vi "Parse REST Device Readings.vi"(3 "error in (no error)":errorcluster, 5 "Reading XML":string="<?xml version=\"1.0\" encoding=\"ISO-8859-1\" standalone=\"no\" ?>\n<methodResponse>\n\n  <params>\n    <param>\n      <value>\n        <struct>\n          <member>\n            <name>status</name>\n            <value>\n              <int>0</int>\n            </value>\n          </member>\n          <member>\n            <name>scaled</name>\n            <value>\n              <double>0.9992975666172701</double>\n            </value>\n          </member>\n          <member>\n            <name>units</name>\n            <value>Torr</value>\n          </member>\n          <member>\n            <name>name</name>\n            <value>e:201vac</value>\n          </member>\n        </struct>\n      </value>\n    </param>\n  </params>\n\n</methodResponse>\n") -> (0 "error out":errorcluster, 1 "Pending":bool, 2 "ACNET Device Readings":T1(array[cluster]))   [LabVIEW 2013]
uses:
  <vilib>/xml/Close Reference(Node).vi
  <vilib>/xml/Close Reference(NdList).vi
  <vilib>/xml/NI_XML.lvlib
  <resource>/objmgr/DOMUserDefRef.rc
panel:
  out "Parse Errors":string
  out "XML Response":string
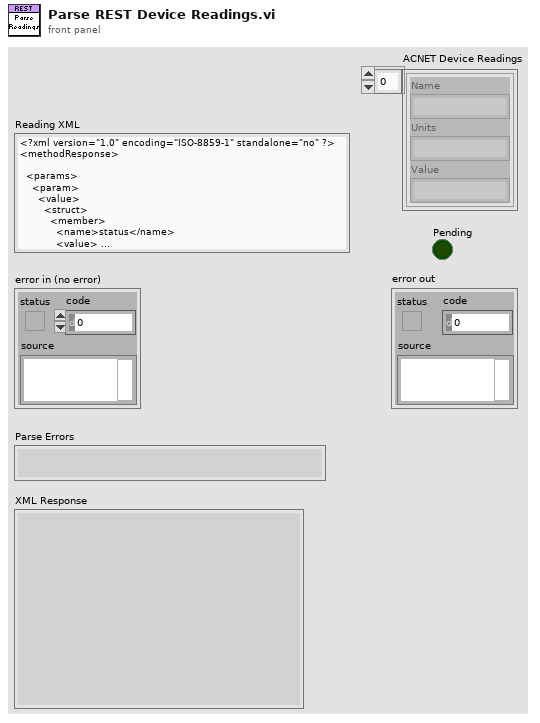
[diagram p1: front panel]
types:
  T1 = cluster{"Name":string, "Units":string, "Value":string}[]
  T2 = cluster{"Name":string, "Units":string, "Value":string}
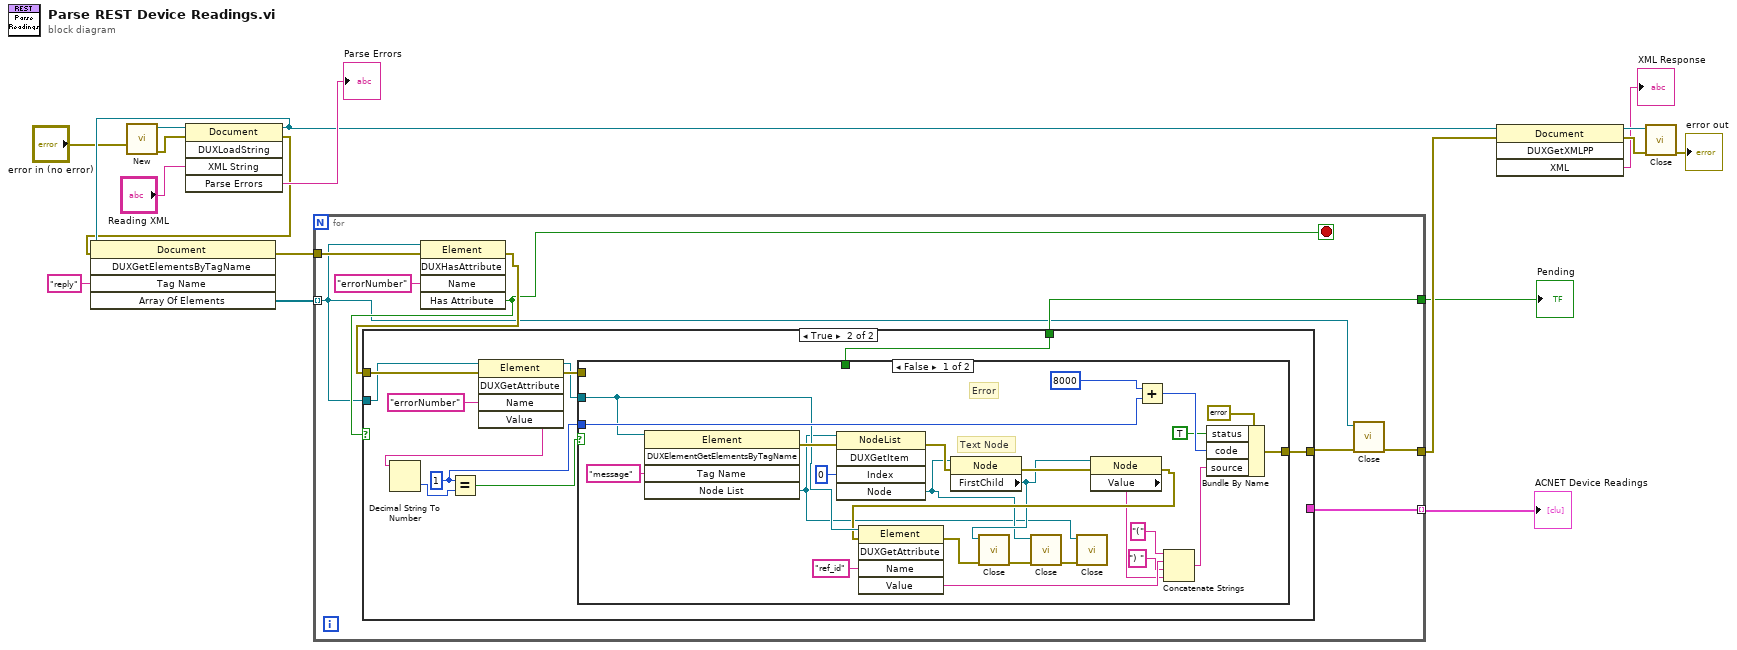
[diagram p0: block diagram]
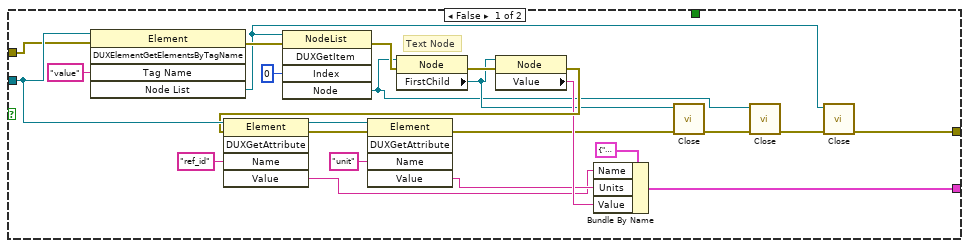
[diagram p2: hidden frame]
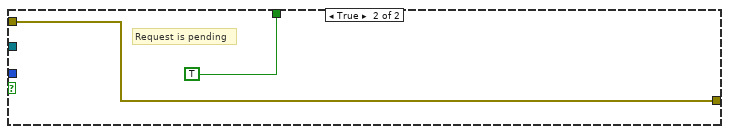
[diagram p3: hidden frame]
diagram:
  n1 = call <vilib>:"New.vi"("error in (no error)"="error in (no error)") -> ("error out"=w13:errorcluster, "DOM document out"=w12:refnum<k20>)  [unwired: 7 in]
  n2 = invoke class="Document" method="DUXLoadString"(reference=w12, error in=w13, "XML String"="Reading XML") -> (reference out=w9:refnum<k20>, error out=w8:errorcluster, "Parse Errors"=→"Parse Errors":string)  [unwired: 2 in, 2 out]
  n3 = invoke class="Document" method="DUXGetElementsByTagName"(reference=w9, error in=w8, "Tag Name"="reply") -> (error out=w6:errorcluster, "Array Of Elements"=w7:refnum<k20>[])  [unwired: 2 in, 3 out]
  n4 = for {
    tunnel: w7 -> [w18] mode=indexing
    tunnel: w6 -> [w26]
    tunnel: [w23] -> w3 mode=indexing
    tunnel: [w21] -> w1
    tunnel: [w20] -> w2
    stop <- w22 stop-if-true
    n5 = invoke class="Element" method="DUXHasAttribute"(reference=w18, error in=w26, "Name"="errorNumber") -> (error out=w24:errorcluster, "Has Attribute"=w22:bool)  [unwired: 2 in, 3 out]
    n6 = case shown="True" w22 {
      tunnel: w18 -> [w48 w58]
      tunnel: w24 -> [w47 w59]
      tunnel: [w33 w54] -> w19
      tunnel: [w34 _] -> w23
      tunnel: [_ w53] -> w21
      frame False {
        # "Text Node"
        n7 = invoke class="Element" method="DUXElementGetElementsByTagName"(reference=w48, error in=w47, "Tag Name"="value") -> (error out=w41:errorcluster, "Node List"=w30:refnum<k20>)  [unwired: 2 in, 3 out]
        n8 = invoke class="NodeList" method="DUXGetItem"(reference=w30, error in=w41, "Index"=0) -> (error out=w39:errorcluster, "Node"=w27:refnum<k20>)  [unwired: 2 in, 3 out]
        n9 = property class="Node"(reference=w27, error in=w39) -> (error out=w49:errorcluster, "FirstChild"=w31:refnum<k20>)  [unwired: 1 out]
        n10 = property class="Node"(reference=w31, error in=w49) -> (error out=w44:errorcluster, "Value"=w37:string)  [unwired: 1 out]
        n11 = invoke class="Element" method="DUXGetAttribute"(reference=w48, error in=w44, "Name"="ref_id") -> (reference out=w43:refnum<k20>, error out=w42:errorcluster, "Value"=w35:string)  [unwired: 2 in, 2 out]
        n12 = invoke class="Element" method="DUXGetAttribute"(reference=w43, error in=w42, "Name"="unit") -> (error out=w32:errorcluster, "Value"=w36:string)  [unwired: 2 in, 3 out]
        n13 = Bundle By Name(cluster=T2 {"Name"="", "Units"="", "Value"=""}, "Name"=w35, "Units"=w36, "Value"=w37) -> (w34:T2)
        n14 = call-poly <vilib>:"Close.vi"("error in (no error)"=w32, "node"=w31) -> ("error out"=w29:errorcluster)  [unwired: 7 in]
        n15 = call-poly <vilib>:"Close.vi"("error in (no error)"=w29, "node"=w27) -> ("error out"=w28:errorcluster)  [unwired: 7 in]
        n16 = call-poly <vilib>:"Close.vi"("error in (no error)"=w28, "node list"=w30) -> ("error out"=w33:errorcluster)  [unwired: 7 in]
      }
      frame True {
        w52 = 1 ("x")
        n17 = invoke class="Element" method="DUXGetAttribute"(reference=w58, error in=w59, "Name"="errorNumber") -> (reference out=w51:refnum<k20>, error out=w55:errorcluster, "Value"=w60:string)  [unwired: 2 in, 2 out]
        n18 = Decimal String To Number(string=w60) -> (number=w57:i32)  [unwired: 2 in, 1 out]
        n19 = Equal?(x=w52, y=w57) -> (x = y?=w56:bool)
        n20 = case shown="False" w56 {
          tunnel: w55 -> [_ w88]
          tunnel: [w83 w88] -> w54
          tunnel: [_ TRUE ("Has Attribute")] -> w53
          tunnel: w52 -> [w76 _]
          tunnel: w51 -> [w74 _]
          frame False {
            # "Text Node"
            # "Error"
            n21 = invoke class="Element" method="DUXElementGetElementsByTagName"(reference=w74, "Tag Name"="message") -> (error out=w80:errorcluster, "Node List"=w62:refnum<k20>)  [unwired: 3 in, 3 out]
            n22 = invoke class="NodeList" method="DUXGetItem"(reference=w62, error in=w80, "Index"=0) -> (error out=w78:errorcluster, "Node"=w63:refnum<k20>)  [unwired: 2 in, 3 out]
            n23 = property class="Node"(reference=w63, error in=w78) -> (error out=w81:errorcluster, "FirstChild"=w66:refnum<k20>)  [unwired: 1 out]
            n24 = property class="Node"(reference=w66, error in=w81) -> (error out=w73:errorcluster, "Value"=w69:string)  [unwired: 1 out]
            n25 = invoke class="Element" method="DUXGetAttribute"(reference=w74, error in=w73, "Name"="ref_id") -> (error out=w65:errorcluster, "Value"=w71:string)  [unwired: 2 in, 3 out]
            n26 = call-poly <vilib>:"Close.vi"("error in (no error)"=w65, "node"=w66) -> ("error out"=w67:errorcluster)  [unwired: 7 in]
            n27 = call-poly <vilib>:"Close.vi"("error in (no error)"=w67, "node"=w63) -> ("error out"=w64:errorcluster)  [unwired: 7 in]
            n28 = call-poly <vilib>:"Close.vi"("error in (no error)"=w64, "node list"=w62) -> ()  [unwired: 7 in, 1 out]
            n29 = Add(x=8000 ("code"), y=w76) -> (x+y=w85:i32)
            n30 = Concatenate Strings("(" ("string"), w71, ") " ("string"), w69) -> (w68:string)
            n31 = Bundle By Name(cluster=errorcluster {"status"=FALSE, "code"=0, "source"=""} ("error out"), "status"=TRUE, "code"=w85, "source"=w68) -> (w83:errorcluster)
          }
          frame True {
            # "Request is pending"
            # "Pending"
          }
        }
      }
    }
    n32 = call-poly <vilib>:"Close.vi"("error in (no error)"=w19, "node"=w18) -> ("error out"=w20:errorcluster)  [unwired: 7 in]
  }
  "ACNET Device Readings" <- w3
  "Pending" <- w1
  n33 = invoke class="Document" method="DUXGetXMLPP"(reference=w9, error in=w2) -> (reference out=w16:refnum<k20>, error out=w17:errorcluster, "XML"=→"XML Response":string)  [unwired: 2 in, 1 out]
  n34 = call-poly <vilib>:"Close.vi"("error in (no error)"=w17, "node"=w16) -> ("error out"=→"error out":errorcluster)  [unwired: 7 in]
